vi "CreateChannels.vi"(8 "error in":errorcluster) -> (0 "error out":errorcluster, 3 "task out":refnum<k21>)   [LabVIEW 2017]
uses:
  <vilib>/DAQmx/configure/timing.llb/DAQmx Timing (Sample Clock).vi
  <vilib>/DAQmx/create/channels.llb/DAQmx Create Channel (AI-Voltage-Basic).vi
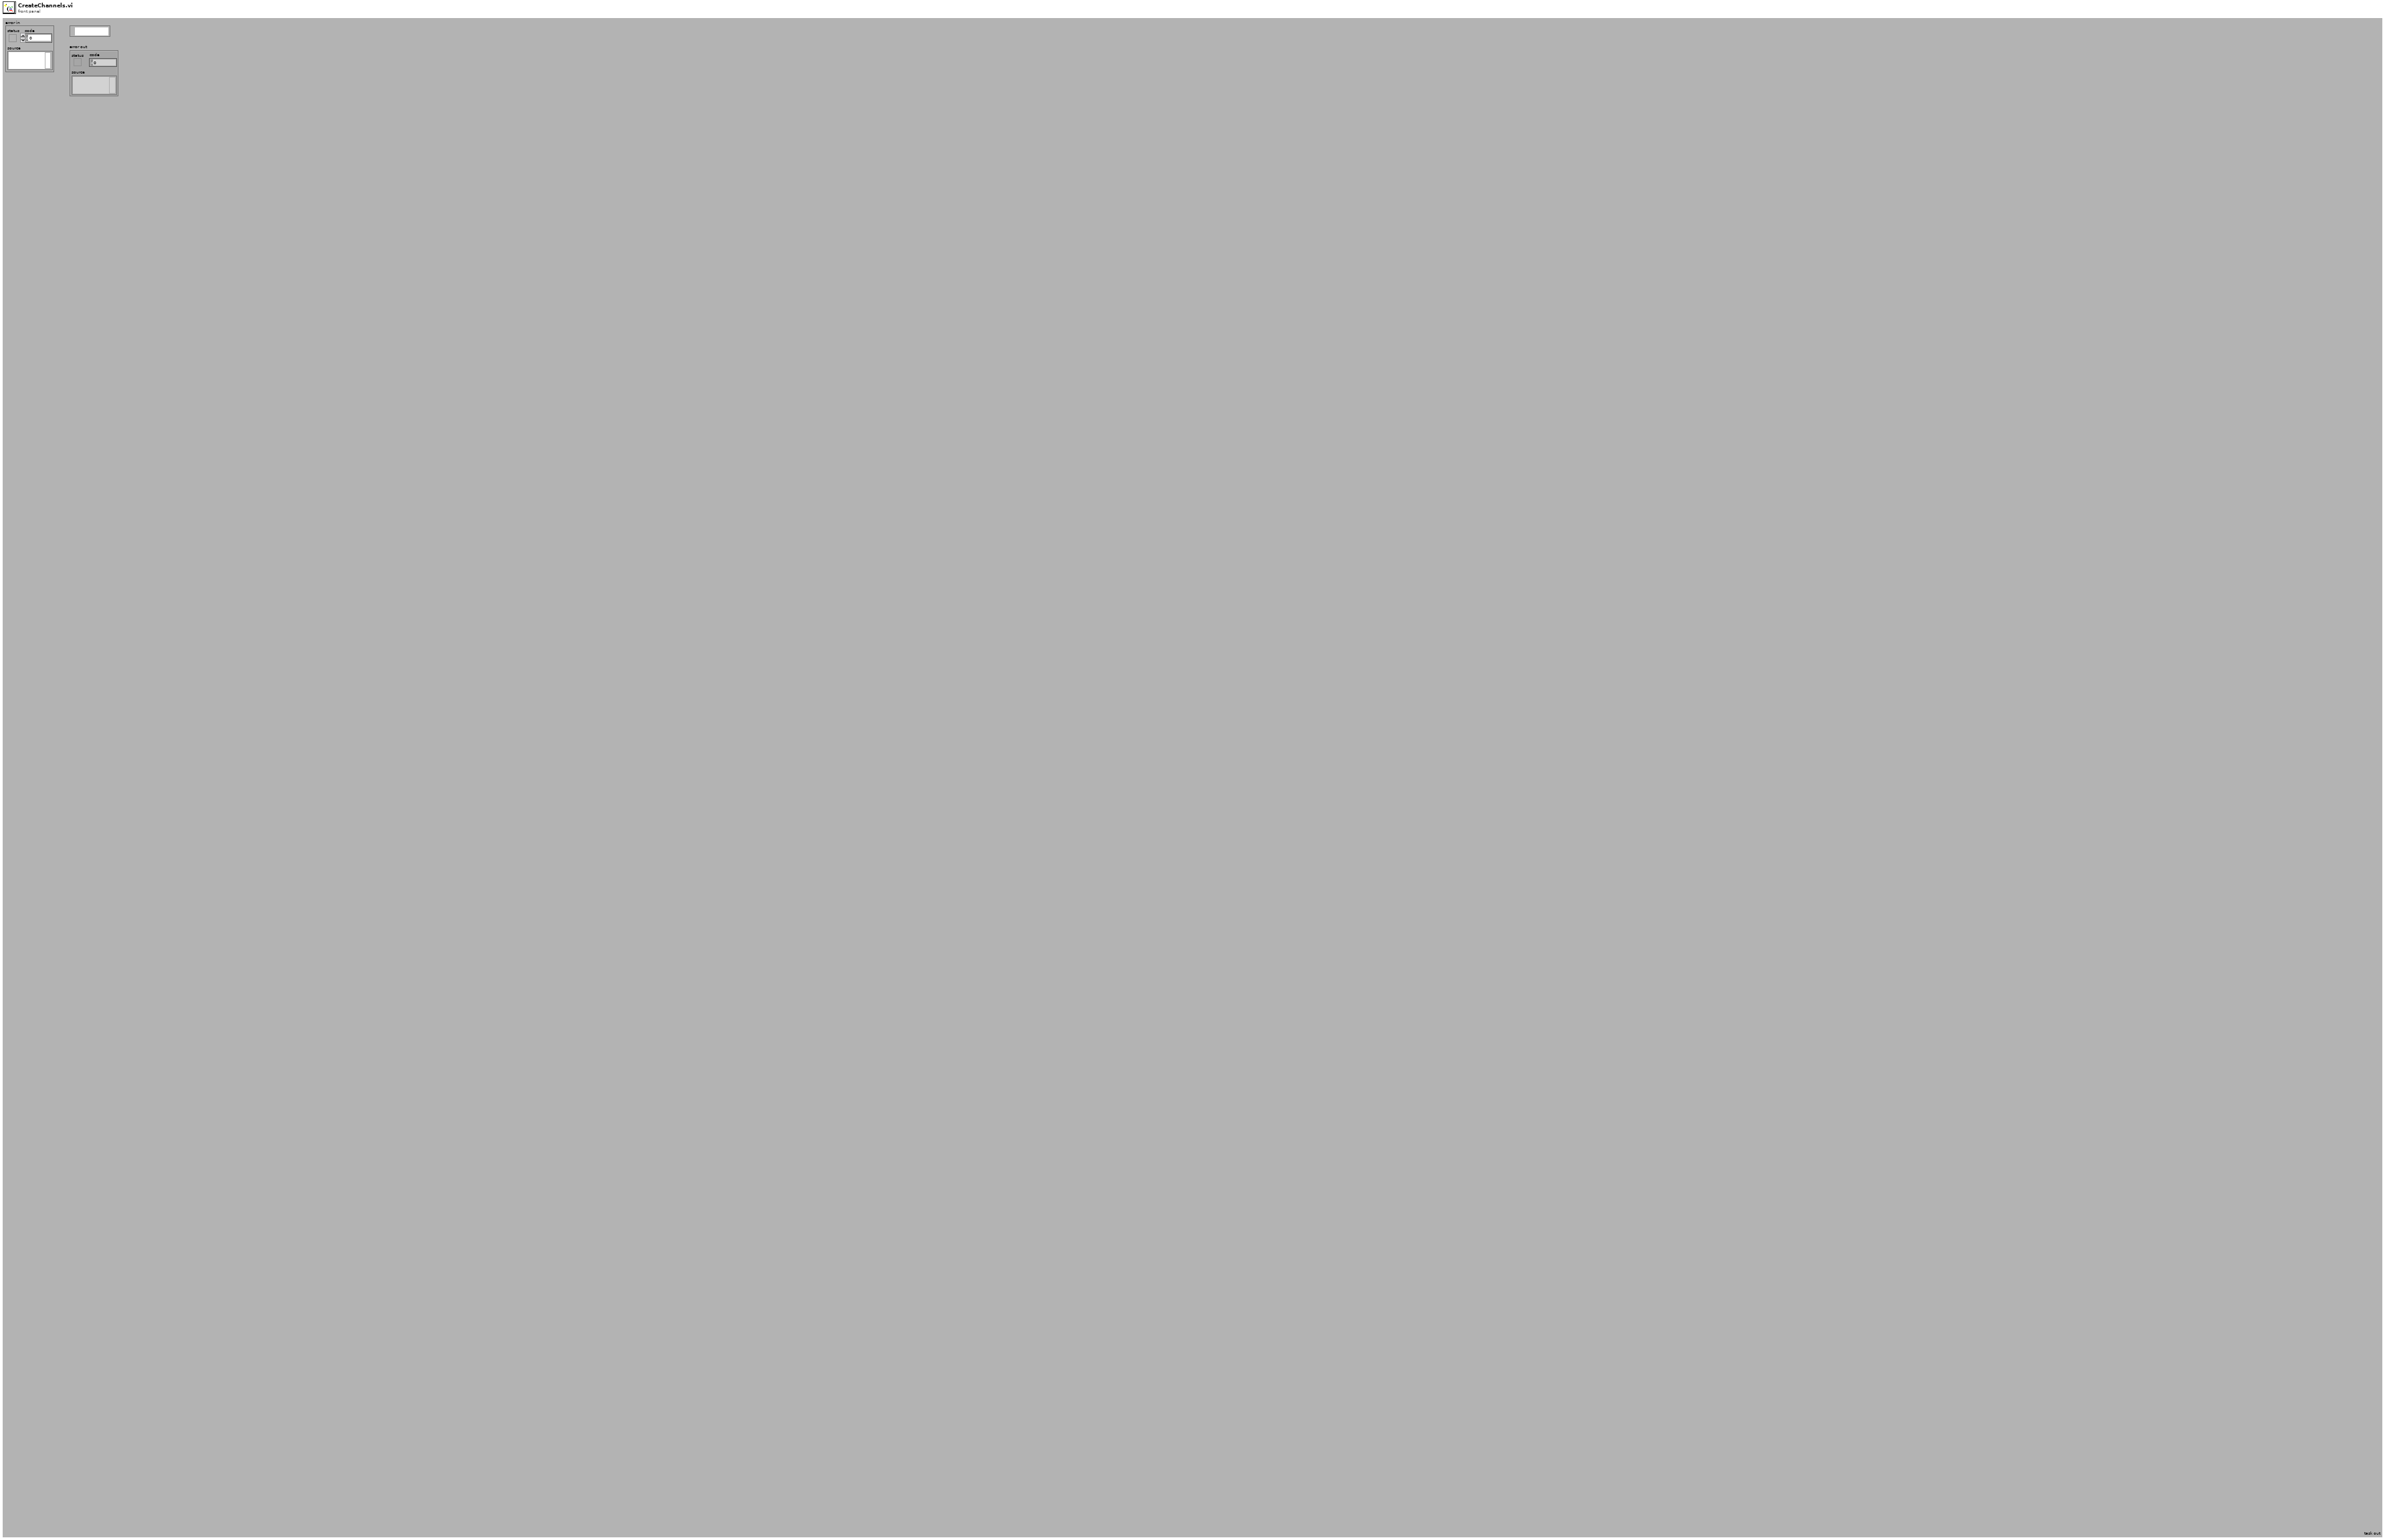
[diagram p1: front panel]
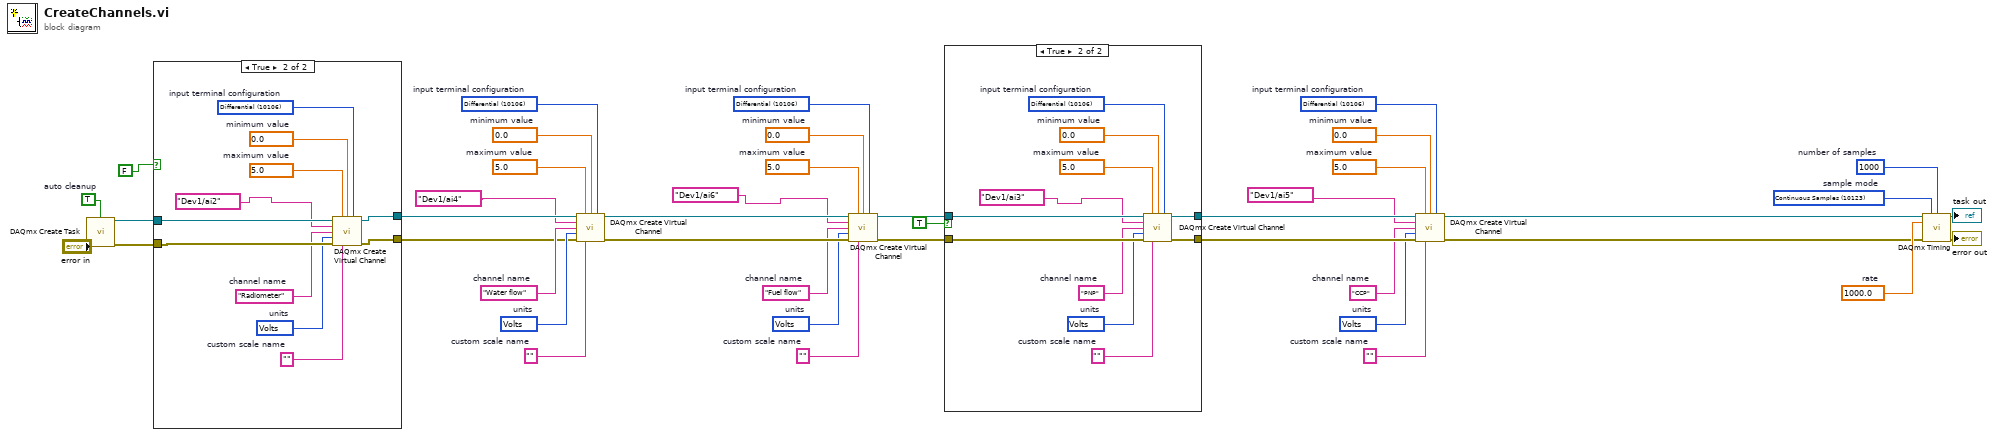
[diagram p0: block diagram]
diagram:
  w6 = 10106 items=["default"=-1, "RSE"=10083, "NRSE"=10078, "Differential"=10106, "Pseudodifferential"=12529]  # input terminal configuration
  w7 = 10348 items=["Volts"=10348, "From Custom Scale"=10065]  # units
  w8 = "Fuel flow"  # channel name
  w9 = ""  # custom scale name
  w10 = 0.0  # minimum value
  w11 = 5.0  # maximum value
  w13 = 10106 items=["default"=-1, "RSE"=10083, "NRSE"=10078, "Differential"=10106, "Pseudodifferential"=12529]  # input terminal configuration
  w14 = 10348 items=["Volts"=10348, "From Custom Scale"=10065]  # units
  w15 = "Water flow"  # channel name
  w17 = ""  # custom scale name
  w18 = 0.0  # minimum value
  w19 = 5.0  # maximum value
  w26 = 10123 items=["Finite Samples"=10178, "Continuous Samples"=10123, "Hardware Timed Single Point"=12522]  # sample mode
  w27 = 1000  # number of samples
  w28 = 1000.0  # rate
  w31 = 10106 items=["default"=-1, "RSE"=10083, "NRSE"=10078, "Differential"=10106, "Pseudodifferential"=12529]  # input terminal configuration
  w32 = 10348 items=["Volts"=10348, "From Custom Scale"=10065]  # units
  w33 = "CCP"  # channel name
  w34 = ""  # custom scale name
  w35 = 0.0  # minimum value
  w36 = 5.0  # maximum value
  w41 = TRUE  # auto cleanup
  n1 = call <vilib>:"DAQmx Create Task.vi"("auto cleanup"=w41, "error in"="error in") -> ("task out"=w25:refnum<k21>, "error out"=w24:errorcluster)  [unwired: 12 in]
  n2 = case shown="True" FALSE {
    tunnel: w25 -> [w44 w55]
    tunnel: w24 -> [w43 w54]
    tunnel: [w44 w47] -> w5
    tunnel: [w43 w46] -> w4
    frame False {
    }
    frame True {
      w53 = 10106 items=["default"=-1, "RSE"=10083, "NRSE"=10078, "Differential"=10106, "Pseudodifferential"=12529]  # input terminal configuration
      w52 = 10348 items=["Volts"=10348, "From Custom Scale"=10065]  # units
      w51 = "Radiometer"  # channel name
      w50 = ""  # custom scale name
      w49 = 0.0  # minimum value
      w48 = 5.0  # maximum value
      n3 = call-poly <vilib>:"DAQmx Create Virtual Channel.vi"("task in"=w55, "maximum value"=w48, "minimum value"=w49, "input terminal configuration"=w53, "physical channels"=tag "Dev1/ai2", "name to assign"=w51, "units"=w52, "error in"=w54, "custom scale name"=w50) -> ("task out"=w47:refnum<k21>, "error out"=w46:errorcluster)  [unwired: 5 in]
    }
  }
  n4 = call-poly <vilib>:"DAQmx Create Virtual Channel.vi"("task in"=w5, "maximum value"=w19, "minimum value"=w18, "input terminal configuration"=w13, "physical channels"=tag "Dev1/ai4", "name to assign"=w15, "units"=w14, "error in"=w4, "custom scale name"=w17) -> ("task out"=w12:refnum<k21>, "error out"=w16:errorcluster)  [unwired: 5 in]
  n5 = call-poly <vilib>:"DAQmx Create Virtual Channel.vi"("task in"=w12, "maximum value"=w11, "minimum value"=w10, "input terminal configuration"=w6, "physical channels"=tag "Dev1/ai6", "name to assign"=w8, "units"=w7, "error in"=w16, "custom scale name"=w9) -> ("task out"=w39:refnum<k21>, "error out"=w40:errorcluster)  [unwired: 5 in]
  n6 = case shown="True" TRUE {
    tunnel: w40 -> [w56 w68]
    tunnel: w39 -> [w57 w67]
    tunnel: [w56 w63] -> w38
    tunnel: [w57 w59] -> w37
    frame False {
    }
    frame True {
      w60 = 10106 items=["default"=-1, "RSE"=10083, "NRSE"=10078, "Differential"=10106, "Pseudodifferential"=12529]  # input terminal configuration
      w61 = 10348 items=["Volts"=10348, "From Custom Scale"=10065]  # units
      w62 = "PNP"  # channel name
      w64 = ""  # custom scale name
      w65 = 0.0  # minimum value
      w66 = 5.0  # maximum value
      n7 = call-poly <vilib>:"DAQmx Create Virtual Channel.vi"("task in"=w67, "maximum value"=w66, "minimum value"=w65, "input terminal configuration"=w60, "physical channels"=tag "Dev1/ai3", "name to assign"=w62, "units"=w61, "error in"=w68, "custom scale name"=w64) -> ("task out"=w59:refnum<k21>, "error out"=w63:errorcluster)  [unwired: 5 in]
    }
  }
  n8 = call-poly <vilib>:"DAQmx Create Virtual Channel.vi"("task in"=w37, "maximum value"=w36, "minimum value"=w35, "input terminal configuration"=w31, "physical channels"=tag "Dev1/ai5", "name to assign"=w33, "units"=w32, "error in"=w38, "custom scale name"=w34) -> ("task out"=w23:refnum<k21>, "error out"=w22:errorcluster)  [unwired: 5 in]
  n9 = call-poly <vilib>:"DAQmx Timing.vi"("task/channels in"=w23, "sample mode"=w26, "samples per channel"=w27, "rate"=w28, "error in"=w22) -> ("task out"=→"task out":refnum<k21>, "error out"=→"error out":errorcluster)  [unwired: 9 in]
